vi "Read OTP header.vi"(5 "Write to file":bool, 7 "selected path":path, 8 "error in (no error)":errorcluster, 9 "reference":refnum<vi>, 10 "OTP values to read":string="0:127/1", 11 "PIC-Device in":refnum<class "PIC-Device.lvclass">) -> (0 "error out":errorcluster, 1 "Array":string[](array[string]), 3 "PIC-Device out":refnum<class "PIC-Device.lvclass">)   [LabVIEW 2020, in "PIC-Device.lvclass"]
uses:
  PIC-Device.lvclass
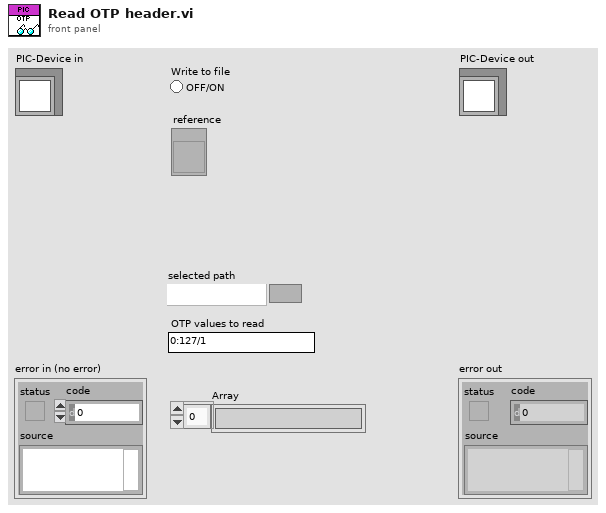
[diagram p1: front panel]
types:
  T1 = typedef "PIC-Device.lvclass/Register to Write.ctl" = cluster{"Register":u32, "Value":u32, "Dev Address":u32, "Physical Adress":u32}
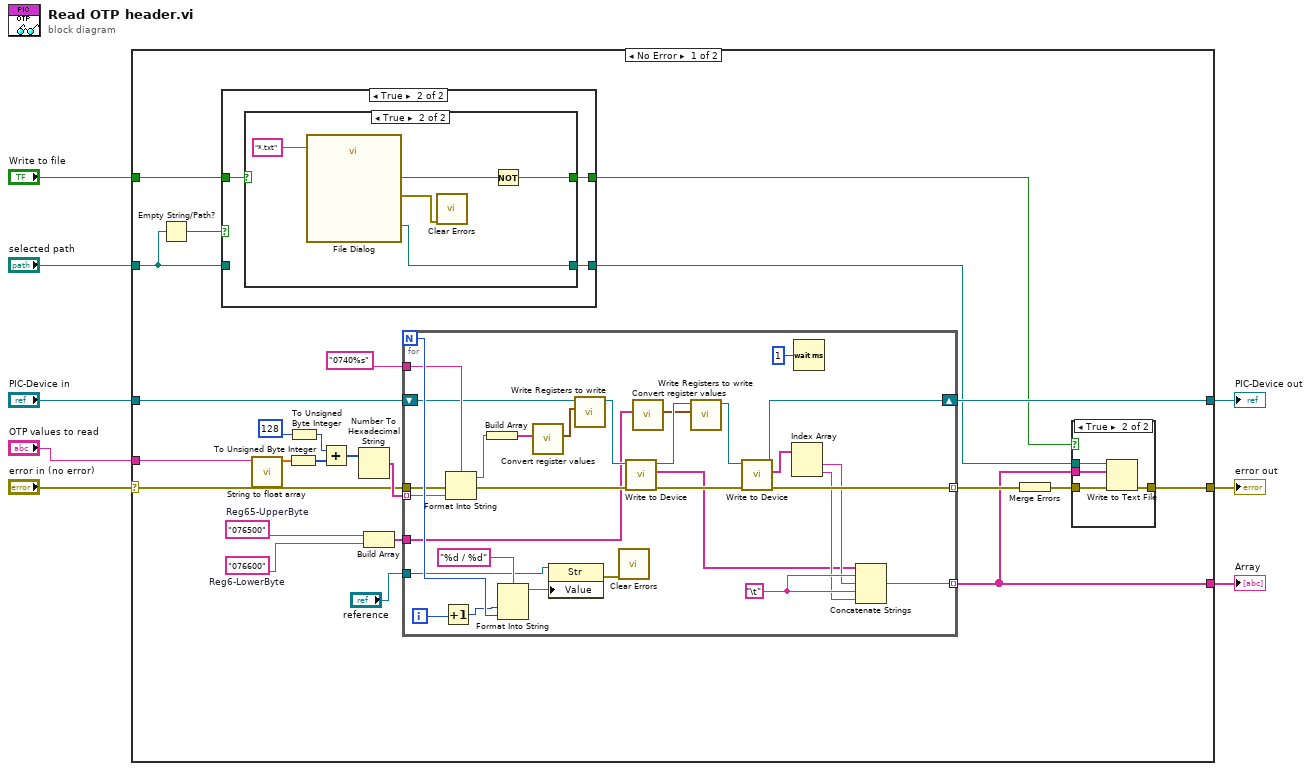
[diagram p0: block diagram]
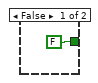
[diagram p3: hidden frame]
diagram:
  n1 = case shown="No Error" "error in (no error)" {
    selector: "error in (no error)" -> [w17 w80]
    tunnel: [w16 w80] -> w7
    tunnel: [w18 w79] -> w5
    tunnel: "PIC-Device in" -> [w19 w79]
    tunnel: "selected path" -> [w12 _]
    tunnel: "Write to file" -> [w9 _]
    tunnel: "OTP values to read" -> [w15 _]
    tunnel: [w14 _] -> w1
    frame No Error {
      w23 = "076600"  # Reg6-LowerByte
      w22 = "076500"  # Reg65-UpperByte
      n2 = Empty String/Path?(string/path=w12) -> (empty?=w13:bool)
      n3 = case shown="True" w13 {
        tunnel: [w34 w37] -> w11
        tunnel: w12 -> [w34 _]
        tunnel: [w33 w36] -> w10
        tunnel: w9 -> [w33 w35]
        frame False {
        }
        frame True {
          n4 = case shown="True" w35 {
            tunnel: [_ w40] -> w37
            tunnel: [FALSE w39] -> w36
            frame False {
            }
            frame True {
              n5 = call "File Dialog"("pattern (all files)"="*.txt") -> ("selected path"=w40:path, "cancelled"=w41:bool, "error out"=w42:errorcluster)  [unwired: 11 in, 1 out]
              n6 = call <vilib>:"Clear Errors.vi"("error in (no error)"=w42) -> ()  [unwired: 5 in, 2 out]
              n7 = Not(x=w41) -> (.not. x?=w39:bool)
            }
          }
        }
      }
      n8 = call "String to float array.vi"("String"=w15) -> ("Array - Numeric"=w27:dbl[])  [unwired: 9 in, 1 out]
      n9 = To Unsigned Byte Integer(number=w27) -> (unsigned 8bit integer=w26:u8[])
      n10 = To Unsigned Byte Integer(number=u8 128) -> (unsigned 8bit integer=w25:u8)
      n11 = Add(x=w25, y=w26) -> (x+y=w24:u8[])
      n12 = Number To Hexadecimal String(2:w24) -> (0:w29:string[])  [unwired: 1 in]
      n13 = Build Array(w22, w23) -> (w31:string[])
      n14 = for {
        N -> [w69]
        tunnel: w17 -> [w56]
        tunnel: [w53] -> w21 mode=indexing
        tunnel: [w71] -> w14 mode=indexing
        tunnel: w29 -> [w57] mode=indexing
        tunnel: "0740%s" -> [w52]
        tunnel: w31 -> [w51]
        shift-right: [w49] -> w18
        shift-left: w19 -> [w50]
        tunnel: "reference" -> [w45]
        i -> [w68]
        w72 = "\t"
        n15 = Increment(x=w68) -> (x+1=w67:i32)
        n16 = Format Into String(format string=w52, error in=w56, w57) -> (resulting string=w60:string, error out=w55:errorcluster)  [unwired: 1 in]
        n17 = Build Array(w60) -> (w61:string[])
        n18 = Format Into String(format string="%d / %d", w67, w69) -> (resulting string=w66:string)  [unwired: 2 in, 1 out]
        n19 = call "Convert register values.vi"("Register strings"=w61) -> ("Register clusters out"=w59:T1[])  [unwired: 9 in, 1 out]
        n20 = property class="Str"(reference=w45, "Value"=w66) -> (error out=w44:errorcluster)  [unwired: 1 in, 1 out]
        n21 = call-dynamic "Write Registers to write.vi"("Registers to write"=w59, "Device in"=w50) -> ("Device out"=w58:refnum<class "PIC-Device.lvclass">)  [unwired: 9 in]
        n22 = call <vilib>:"Clear Errors.vi"("error in (no error)"=w44) -> ()  [unwired: 5 in, 2 out]
        n23 = call-dynamic "Write to Device.vi"("error in (no error)"=w55, "Device in"=w58) -> ("error out"=w54:errorcluster, "Return"=w46:string[], "Device out"=w65:refnum<class "PIC-Device.lvclass">)  [unwired: 7 in]
        n24 = call "Convert register values.vi"("Register strings"=w51) -> ("Register clusters out"=w62:T1[])  [unwired: 9 in, 1 out]
        n25 = call-dynamic "Write Registers to write.vi"("Registers to write"=w62, "Device in"=w65) -> ("Device out"=w63:refnum<class "PIC-Device.lvclass">)  [unwired: 9 in]
        n26 = call-dynamic "Write to Device.vi"("error in (no error)"=w54, "Device in"=w63) -> ("error out"=w53:errorcluster, "Return"=w64:string[], "Device out"=w49:refnum<class "PIC-Device.lvclass">)  [unwired: 7 in]
        n27 = Index Array(array=w64) -> (element #1=w48:string, element #2=w47:string)  [unwired: 2 in]
        n28 = Wait (ms)(milliseconds to wait=u32 1) -> ()  [unwired: 1 out]
        n29 = Concatenate Strings(w46, w72, w48, w72, w47) -> (w71:string)
      }
      n30 = Merge Errors(w21) -> (w32:errorcluster)
      n31 = case shown="True" w10 {
        tunnel: [w74 w78] -> w16
        tunnel: w14 -> [_ w77]
        tunnel: w11 -> [_ w76]
        tunnel: w32 -> [w74 w75]
        frame False {
        }
        frame True {
          n32 = Write to Text File(file (use dialog)=w76, text=w77, error in=w75) -> (error out=w78:errorcluster)  [unwired: 1 in, 2 out]
        }
      }
    }
    frame Error {
    }
  }
  "error out" <- w7
  "PIC-Device out" <- w5
  "Array" <- w1
